vi "SetQControl.vi"(8 "error in":T1, 10 "Feedback":sgl=-inf, 11 "Phase":sgl=-inf format="%#_g deg") -> (0 "error out":T1, 2 "Feedback out":sgl, 3 "Phase":sgl format="%#_g deg")   [LabVIEW 2016]
doc: "This VI sets the 'Phase' in degrees between -180° and +180° and the 'Feedback' between 0 and 1 for the Q Control. By passing -Inf as input values, the corresponding parameter(s) will be read out."
uses:
  Controls/Error_Out.ctl
  Files_ASC500/DLL/ASC500_RemoteControlV27.dll
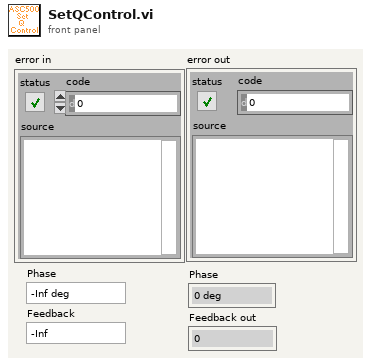
[diagram p1: front panel]
types:
  T1 = typedef "Error_Out.ctl" = errorcluster
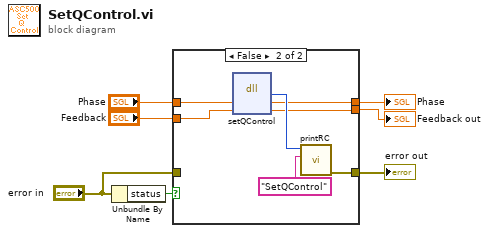
[diagram p0: block diagram]
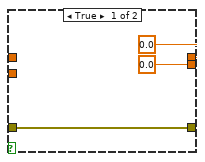
[diagram p2: hidden frame]
diagram:
  n1 = Unbundle By Name("error in") -> ("status"=w7:bool)
  n2 = case shown="False" w7 {
    tunnel: [w10 w15] -> w6
    tunnel: "Phase" -> [_ w17]
    tunnel: "Feedback" -> [_ w16]
    tunnel: "error in" -> [w10 _]
    tunnel: [sgl 0.0 ("Phase") w12] -> w2
    tunnel: [sgl 0.0 ("Feedback") w11] -> w1
    frame True {
    }
    frame False {
      n3 = dll-call lib="G:/SCMOperations/Share/ELE/Produkt Information/ASC500/04 Remote Control/02 development versions/2018Nov06/Files_ASC500/DLL/ASC500_RemoteControlV27.dll" fn="setQControl"("Phase"=w17, "Feedback"=w16) -> ("return type"=w14:i32, "Phase"=w12:sgl, "Feedback"=w11:sgl)  [unwired: 3 in, 2 out]
      n4 = call "printRC.vi"("additional information"="SetQControl", "RC"=w14) -> ("error out"=w15:T1)  [unwired: 9 in]
    }
  }
  "error out" <- w6
  "Phase" <- w2
  "Feedback out" <- w1
